vi "edittest save new sequence.vi"(8 "error in (no error)":errorcluster, 9 "Sequence Fields":T1[](array[typedef]), 10 "Sequence Record In":T4, 11 "Connection Refnum":T5) -> (0 "error out":errorcluster, 2 "Sequence Record":T4, 3 "Connection Refnum":T5)   [LabVIEW 2011]
uses:
  SI.LIB/ODBC/SQL Controls/Connection Refnum.ctl
  server/database/Sequences/Sequence Record.ctl
  server/database/Fields/Field Record.ctl
  server/database/Fields/Field DataTypes.ctl
  server/database/Fields/Field NextItem.ctl
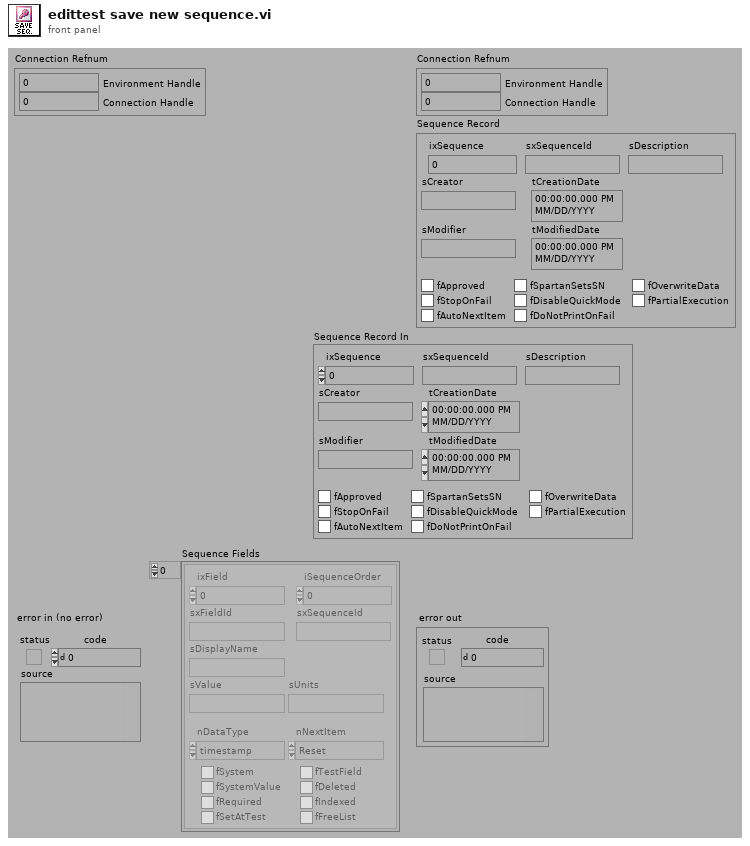
[diagram p1: front panel]
types:
  T1 = typedef "Field Record.ctl" = cluster{"ixField":i32, "iSequenceOrder":i32, "sxFieldId":string, "sxSequenceId":string, "sDisplayName":string, "sValue":string, "sUnits":string, "nDataType":T2, "nNextItem":T3, "fSystem":bool, "fSystemValue":bool, "fRequired":bool, "fSetAtTest":bool, "fTestField":bool, "fDeleted":bool, "fIndexed":bool, "fFreeList":bool}
  T2 = typedef "Field DataTypes.ctl" = enum32{"text", "numeric", "list", "timestamp", "boolean"}
  T3 = typedef "Field NextItem.ctl" = enum32{"Reset", "Retain", "Auto-Increment"}
  T4 = typedef "Sequence Record.ctl" = cluster{"ixSequence":i32, "sxSequenceId":string, "sDescription":string, "sCreator":string, "tCreationDate":timestamp, "sModifier":string, "tModifiedDate":timestamp, "fApproved":bool, "fSpartanSetsSN":bool, "fOverwriteData":bool, "fStopOnFail":bool, "fDisableQuickMode":bool, "fPartialExecution":bool, "fAutoNextItem":bool, "fDoNotPrintOnFail":bool}
  T5 = typedef "Connection Refnum.ctl" = cluster{"Environment Handle":i32, "Connection Handle":i32}
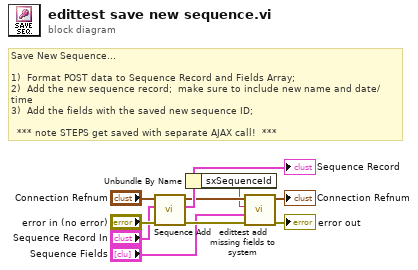
[diagram p0: block diagram]
diagram:
  # "Save New Sequence...\n\n1)  Format POST data to Sequence Record and Fields Array;\n2)  Add the new sequence record;  make sure to include new name and date/time\n3)  Add the fields with the saved new sequence ID;\n\n  *** note STEPS get saved with separate AJAX call!  ***"
  n1 = call "Sequence Add.vi"("error in (no error)"="error in (no error)", "Sequence Record"="Sequence Record In", "Connection Refnum"="Connection Refnum") -> ("error out"=w8:errorcluster, "New Sequence Record"=w10:T4, "Connection Refnum"=w9:T5)  [unwired: 6 out]
  "Sequence Record" <- w10
  n2 = Unbundle By Name(w10) -> ("sxSequenceId"=w5:string)
  n3 = call "edittest add missing fields to system.vi"("error in (no error)"=w8, "Fields"="Sequence Fields", "sxSequenceId (\"\")"=w5, "Connection Refnum"=w9) -> ("error out"=→"error out":errorcluster, "Connection Refnum"=→"Connection Refnum":T5)  [unwired: 6 out]
